vi "Proceed Stop Msg.vi"(8 "priority":i32, 9 "Actor Framework:Stop Msg":refnum<class "Stop Msg.lvclass">, 10 "Caller Enqueuer":refnum<class "Message Enqueuer.lvclass">, 11 "Proxy in":refnum<class "Proxy.lvclass">) -> (0 "error out":errorcluster, 3 "Actor out":refnum<class "Actor.lvclass">)   [LabVIEW 2014, in "Proxy.lvlib" / "Proxy.lvclass"]
uses:
  Proxy.lvclass
  <vilib>/ActorFramework/Message Enqueuer/Message Enqueuer.lvclass
  <vilib>/ActorFramework/Stop Msg/Stop Msg.lvclass
  <vilib>/ActorFramework/Actor/Actor.lvclass
  <vilib>/ActorFramework/Actor/Actor.lvclass/Actor.ctl
  <vilib>/ActorFramework/Message Enqueuer/Message Enqueuer.lvclass/Message Enqueuer.ctl
  <vilib>/ActorFramework/Message Enqueuer/Init from Existing Queue.vi
  <vilib>/ActorFramework/Message Enqueuer/Enqueue.vi
  <vilib>/ActorFramework/Message Priority Queue/Priority Enqueue.vi
  Proxy Messages/Proxy Stop Msg/Proxy Stop Msg.lvclass
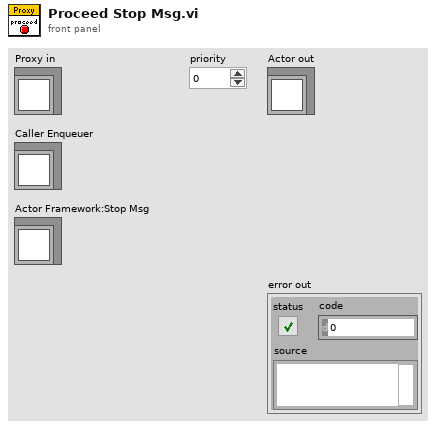
[diagram p1: front panel]
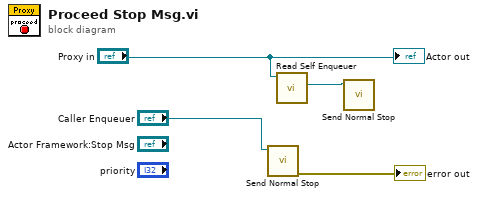
[diagram p0: block diagram]
diagram:
  n1 = call <vilib>:"Send Normal Stop.vi"("Message Enqueuer"="Caller Enqueuer") -> ("error out"=→"error out":errorcluster)  [unwired: 10 in]
  n2 = call <vilib>:"Read Self Enqueuer.vi"("Actor"="Proxy in") -> ("Self Enqueuer"=w3:refnum<class "Message Enqueuer.lvclass">)  [unwired: 10 in]
  n3 = call <vilib>:"Send Normal Stop.vi"("Message Enqueuer"=w3) -> ()  [unwired: 10 in, 1 out]
  "Actor out" <- "Proxy in"
